vi "Unregister for Waveform Data Events (CDB).vi"(8 "error in (no error)":errorcluster, 11 "registered waveform data event (CDB)":T1) -> (0 "error out":errorcluster)   [LabVIEW 2020, in "NI_VS Waveform Streaming Interface.lvlib"]
doc: "Unregisters all waveform data events associated with the event registration refnum. Event structures that use this event registration refnum no longer receive any events. Wire data to the <B>registered waveform data event (DBL)</B> input to determine the polymorphic instance to use or manually select the instance."
uses:
  <vilib>/NI VeriStand/Execution/WaveformStreaming/NI_VS Waveform Streaming Interface.lvlib
  <vilib>/NI VeriStand/Execution/WaveformStreaming/Registered Waveform Streams Data Event Refnum (CDB).ctl
  <vilib>/NI VeriStand/Execution/WaveformStreaming/Waveform Data Watcher Event Data (CDB).ctl
  <vilib>/NI VeriStand/Execution/WaveformStreaming/WaveformStreamSpecification.ctl
  NationalInstruments.VeriStand.ClientAPI
  <vilib>/NI VeriStand/Execution/WaveformStreaming/WaveformDataWatcherCDB.ctl
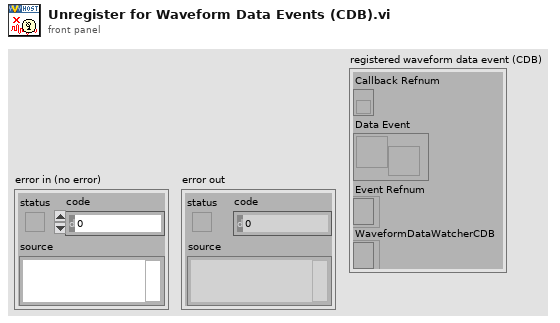
[diagram p1: front panel]
types:
  T1 = typedef "NI_VS Waveform Streaming Interface.lvlib/Registered Waveform Streams Data Event Refnum (CDB).ctl" = cluster{"Callback Refnum":refnum<k27>, "Data Event":refnum<user-event>, "Event Refnum":refnum<event-registration>, "WaveformDataWatcherCDB":T2}
  T2 = typedef "NI_VS Waveform Streaming Interface.lvlib/WaveformDataWatcherCDB.ctl" = refnum<k24>
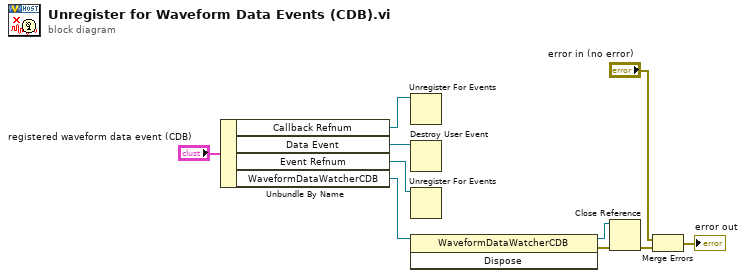
[diagram p0: block diagram]
diagram:
  n1 = Unbundle By Name("registered waveform data event (CDB)") -> ("Callback Refnum"=w9:refnum<k27>, "Data Event"=w8:refnum<user-event>, "Event Refnum"=w7:refnum<event-registration>, "WaveformDataWatcherCDB"=w6:T2)
  n2 = Unregister For Events(event registration refnum=w9) -> ()  [unwired: 1 in, 1 out]
  n3 = Destroy User Event(user event=w8) -> ()  [unwired: 1 in, 1 out]
  n4 = Unregister For Events(event registration refnum=w7) -> ()  [unwired: 1 in, 1 out]
  n5 = invoke class="WaveformDataWatcherCDB" method="Dispose"(reference=w6) -> (reference out=w4:T2, error out=w5:errorcluster)  [unwired: 2 in, 1 out]
  n6 = Close Reference(reference=w4, error in (no error)=w5) -> (error out=w2:errorcluster)
  n7 = Merge Errors("error in (no error)", w2) -> (→"error out":errorcluster)
